vi "ke37xx Configure RTD.vi"(0 "VISA Resource Name":refnum<visa-resource-name>, 5 "Alpha (0.00385)":dbl=0.00385 min=0.0 max=0.1 format="%#_7g", 7 "Beta (0.111)":dbl=0.111 min=0.0 max=1.0 format="%#_7g", 9 "Delta (1.507)":dbl=1.507 min=0.0 max=5.0 format="%#_7g", 11 "error in (no error)":errorcluster, 12 "Zero (100)":dbl=100.0 min=0.0 max=10000.0 format="%#_7g", 13 "3-Wire RTD Type (0: PT100)":T1(ring), 14 "4-Wire RTD Type (0: PT100)":T1(ring)) -> (4 "VISA Resource Name Out":refnum<visa-resource-name>, 15 "error out":errorcluster)   [LabVIEW 2009, in "Keithley 3700 Series.lvlib"]
doc: "This VI allows you to configure various aspects of the RTD used for temperature measurements."
uses:
  <instrlib>/Keithley 3706/Keithley 3700 Series.lvlib
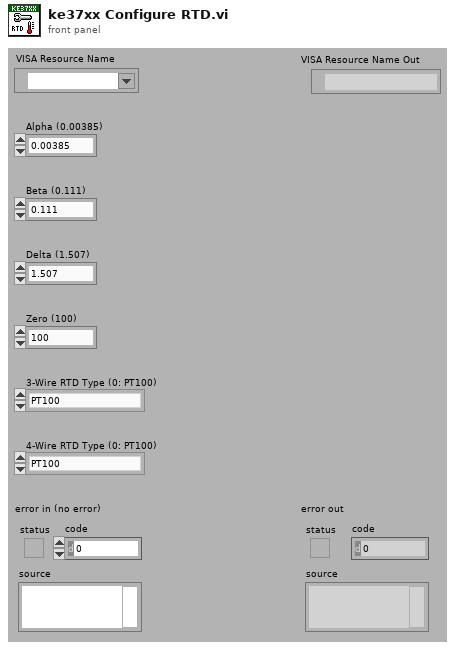
[diagram p1: front panel]
types:
  T1 = enum16{"PT100", "D100", "F100", "PT385", "PT3916", "User"}
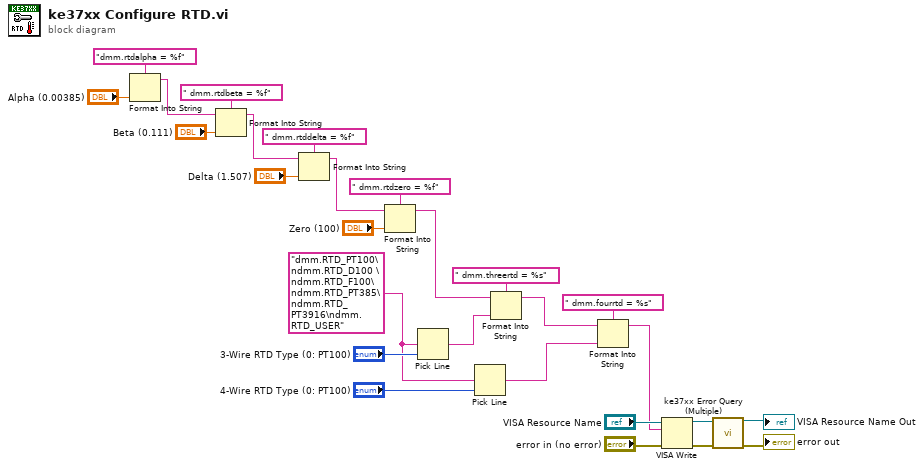
[diagram p0: block diagram]
diagram:
  w16 = "dmm.RTD_PT100\ndmm.RTD_D100 \ndmm.RTD_F100\ndmm.RTD_PT385\ndmm.RTD_PT3916\ndmm.RTD_USER"
  n1 = Format Into String(format string="dmm.rtdalpha = %f" ("write buffer"), "Alpha (0.00385)") -> (resulting string=w7:string)  [unwired: 2 in, 1 out]
  n2 = Format Into String(format string=" dmm.rtdbeta = %f" ("write buffer"), initial string=w7, "Beta (0.111)") -> (resulting string=w5:string)  [unwired: 1 in, 1 out]
  n3 = Format Into String(format string=" dmm.rtddelta = %f" ("write buffer"), initial string=w5, "Delta (1.507)") -> (resulting string=w3:string)  [unwired: 1 in, 1 out]
  n4 = Format Into String(format string=" dmm.rtdzero = %f" ("write buffer"), initial string=w3, "Zero (100)") -> (resulting string=w1:string)  [unwired: 1 in, 1 out]
  n5 = Pick Line(multi-line string=w16, line index="3-Wire RTD Type (0: PT100)") -> (output string=w20:string)  [unwired: 1 out]
  n6 = Pick Line(multi-line string=w16, line index="4-Wire RTD Type (0: PT100)") -> (output string=w19:string)  [unwired: 1 out]
  n7 = Format Into String(format string=" dmm.threertd = %s" ("write buffer"), initial string=w1, w20) -> (resulting string=w14:string)  [unwired: 1 in, 1 out]
  n8 = Format Into String(format string=" dmm.fourrtd = %s" ("write buffer"), initial string=w14, w19) -> (resulting string=w13:string)  [unwired: 1 in, 1 out]
  n9 = VISA Write(VISA resource name="VISA Resource Name", write buffer=w13, error in (no error)="error in (no error)") -> (VISA resource name out=w23:refnum<visa-resource-name>, error out=w22:errorcluster)  [unwired: 1 out]
  n10 = call <instrlib>:"ke37xx Error Query (Multiple).vi"("VISA resource name"=w23, "error in (no error)"=w22) -> ("VISA resource name out"=→"VISA Resource Name Out":refnum<visa-resource-name>, "error out"=→"error out":errorcluster)  [unwired: 12 out]
